vi "MSEncoder SubVI WfmCodeGen_AuxScan.vi"(0 "MSEncoder in":refnum<class "MSEncoder.lvclass">=refnum, 1 "Scan time":ext=0.1, 2 "Pulse1 Amp":ext=-0.55, 3 "mz0":ext=608.9080247841045691, 4 "Amp ramp rate":ext=-0.0, 5 "Pulse2 Amp":ext=0.55, 6 "Start conj #":u32, 7 "Scan rate":ext=-0.0, 8 "Beta scale":ext=1.0, 9 "Wfm type":u64=2, 10 "MathieuEqParame":T1={"mz(Th)"=608.9080247841045691, "Amp(V)"=300.0, "Freq(Hz)"=301269.66536045074, "Beta"=0.39999999999999986, "r_0 (mm)"=10.0, "z_0 (mm)"=7.07106781187} {"Freq(Hz)" format="%#_2g"; "Amp(V)" format="%#.2g"; "mz(Th)" format="%#.2g"}, 11 "Amp0":ext, 13 "TotalAuxCyc#":ext=1.0) -> (17 "WfmCode":u64[](array[numeric]), 19 "error out":errorcluster)   [LabVIEW 2018, in "MSEncoder.lvclass"]
uses:
  MSEncoder.lvclass
  PublicSubVI/Ctl/MathieuEqParam.ctl
  MSEncoder.lvclass/MSEncoder.ctl
panel:
  in  "High Res":bool
  out "start conj":u64[](array[numeric])
  out "RF Cycle":u64[](array[numeric])
  out "decimated array":u64[](array[numeric])
  in  "Interrupt":bool
  out "Aux Scan":cluster{"Scan time":ext, "Actual Freq":dbl}[](graph)
  out "Progress":dbl(slide)=-1.0 scale=0.0..0.1
  out "PriRF.Decyc":u32=32348584
  out "CrntConj.CycDiff":u64[](array[numeric])=[2147483648]
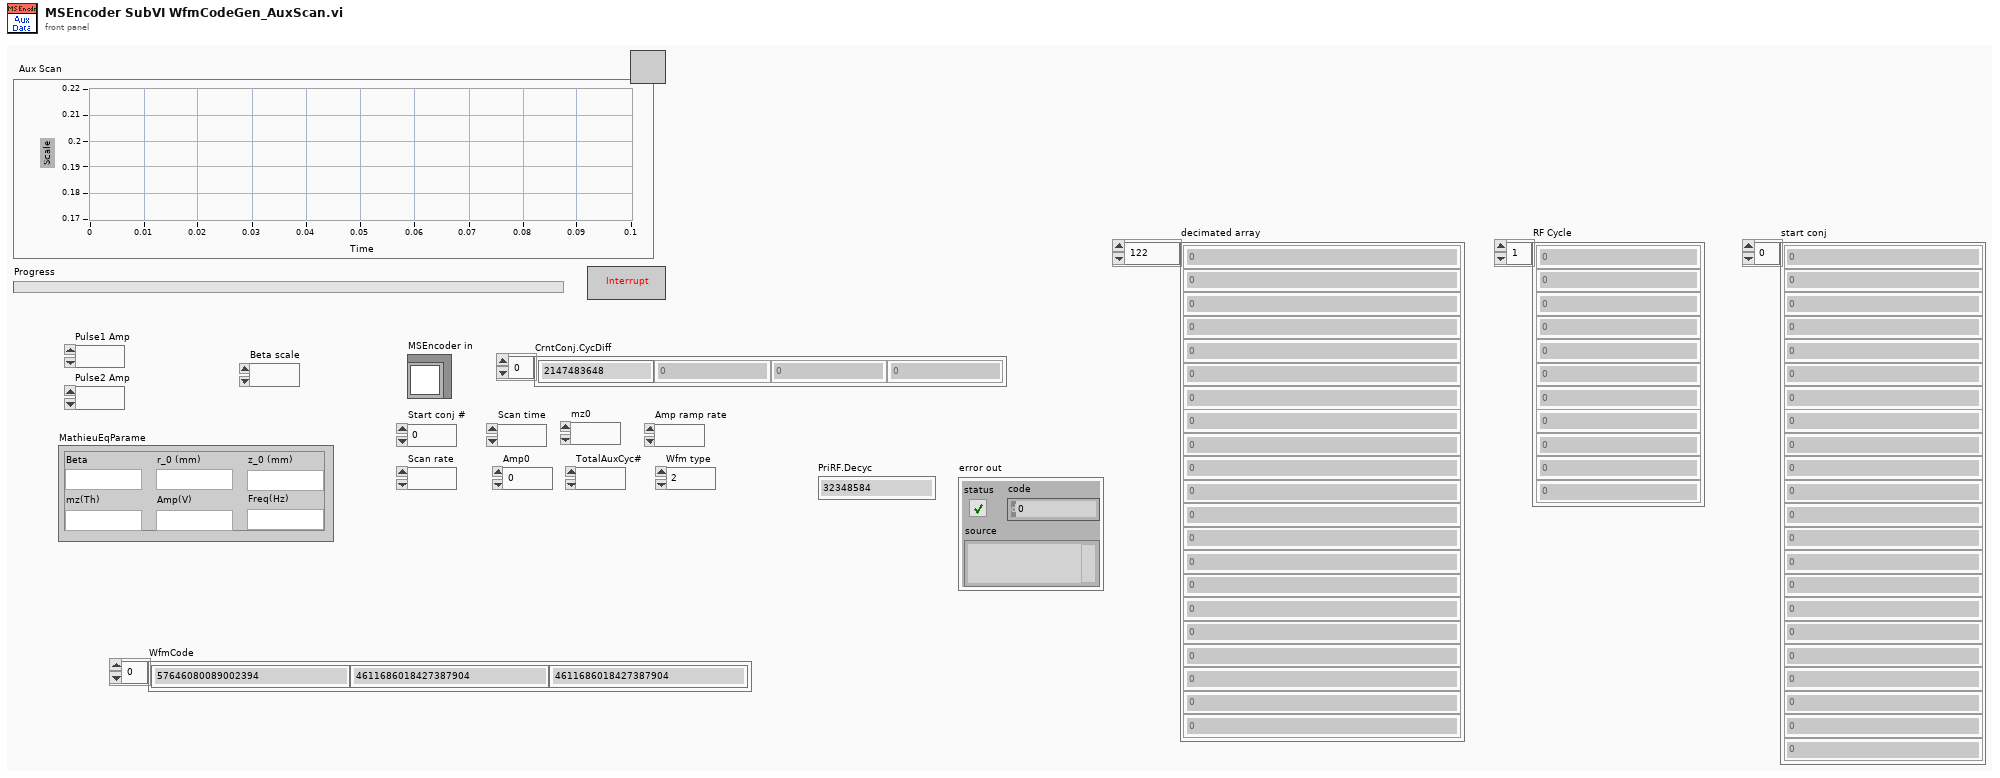
[diagram p1: front panel]
types:
  T1 = typedef "MathieuEqParam.ctl" = cluster{"mz(Th)":ext, "Amp(V)":ext, "Freq(Hz)":ext, "Beta":ext, "r_0 (mm)":ext, "z_0 (mm)":ext}
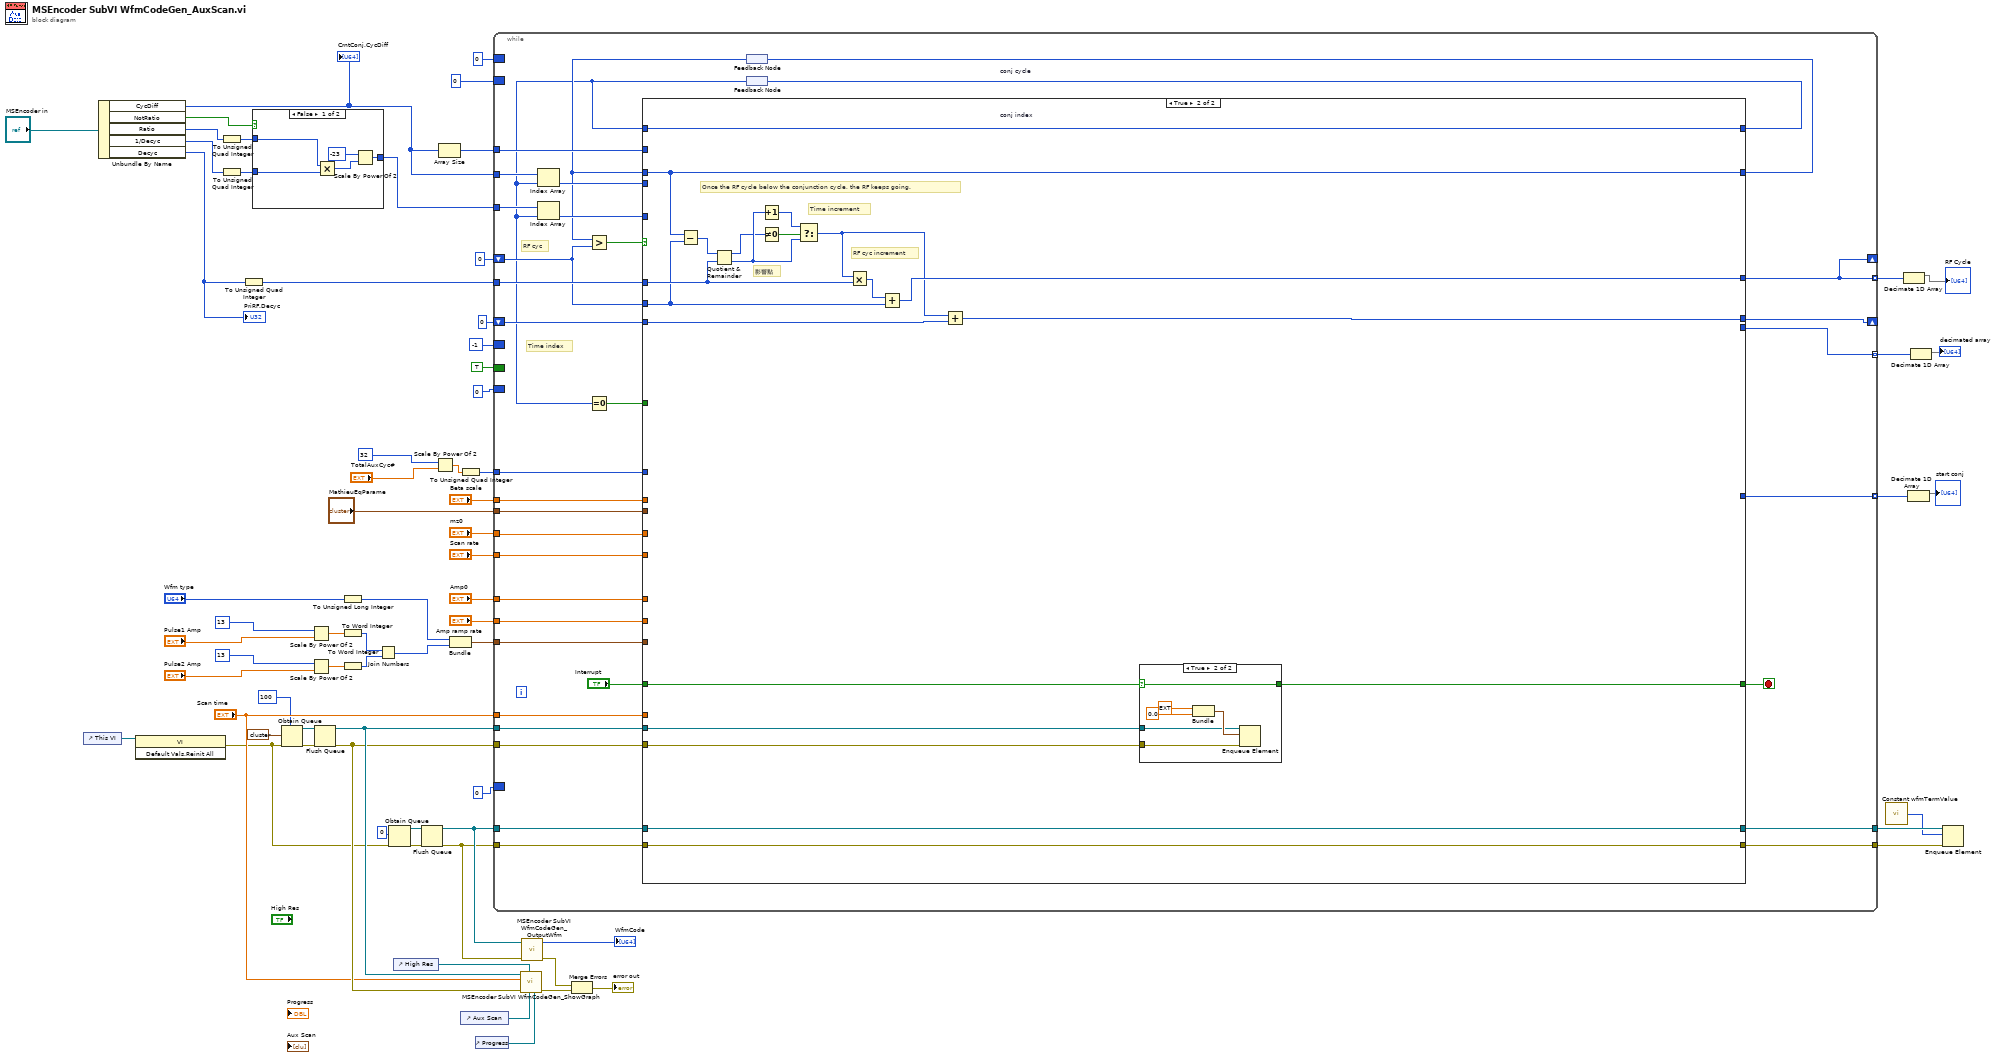
[diagram p0: block diagram]
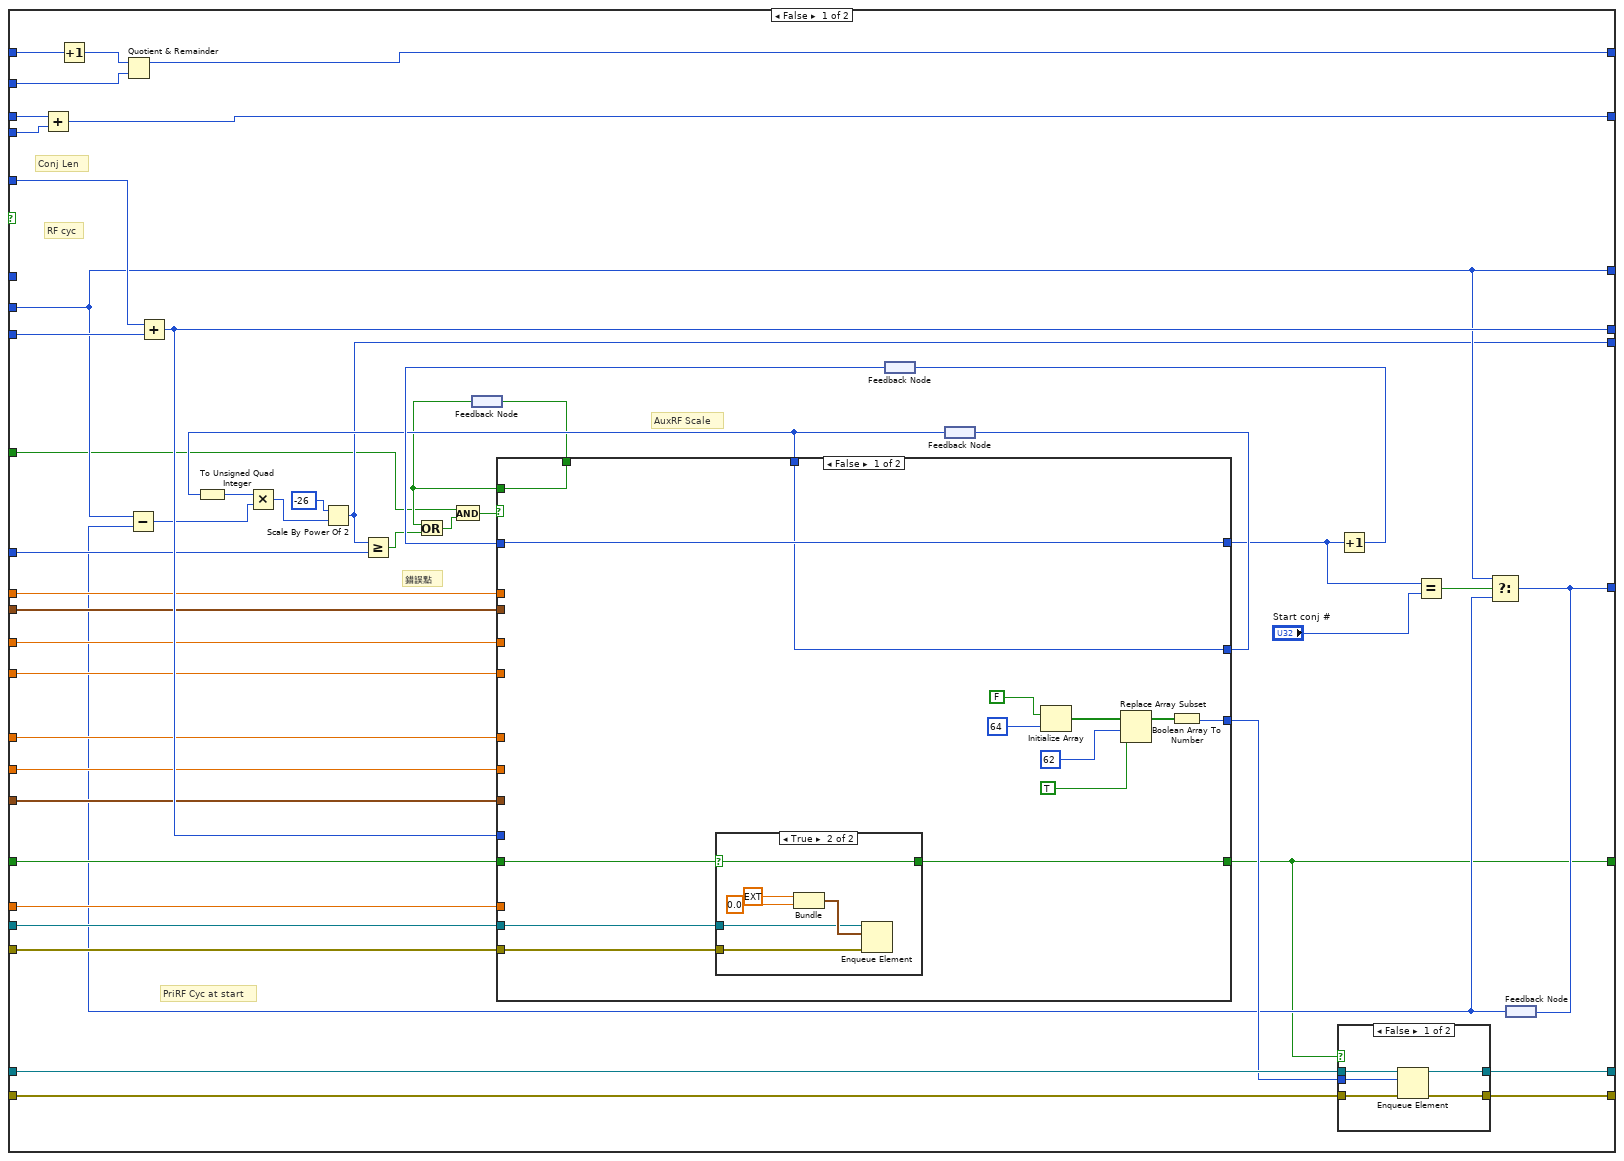
[diagram p3: hidden frame]
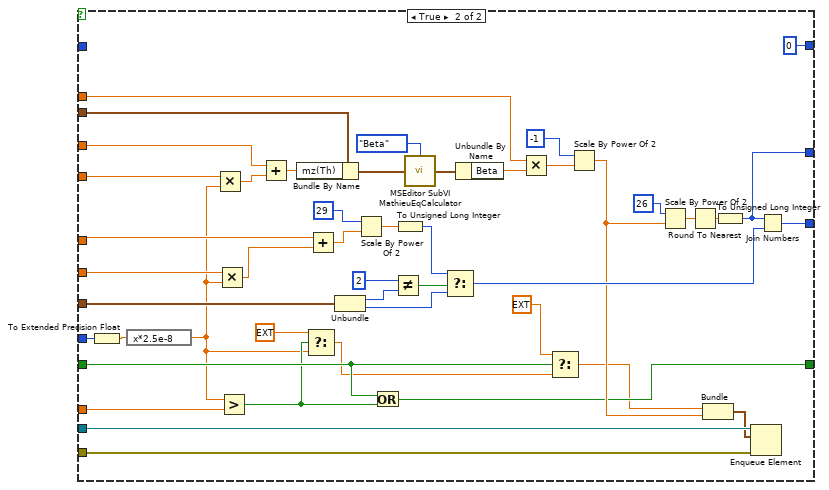
[diagram p6: hidden frame]
diagram:
  n1 = control-ref of="This VI"() -> (w9:refnum<vi>)
  n2 = Unbundle By Name("MSEncoder in") -> ("CycDiff"=w56:u64[], "NotRatio"=w40:bool, "Ratio"=w68:u16[], "1/Decyc"=w69:u32, "Decyc"=w71:u32)
  "CrntConj.CycDiff" <- w56
  "PriRF.Decyc" <- w71
  n3 = invoke class="VI" method="Default Vals.Reinit All"(reference=w9) -> (error out=w8:errorcluster)  [unwired: 2 in, 2 out]
  n4 = To Unsigned Quad Integer(1:w68) -> (0:w70:u64[])
  n5 = To Unsigned Quad Integer(1:w69) -> (0:w54:u64)
  n6 = To Unsigned Quad Integer(1:w71) -> (0:w53:u64)
  n7 = case shown="False" w40 {
    tunnel: w70 -> [w74 w77]
    tunnel: [w73 w77] -> w57
    tunnel: w54 -> [w72 _]
    frame False {
      n8 = Multiply(x=w74, y=w72) -> (x*y=w75:u64[])
      n9 = Scale By Power Of 2(n=i16 -23, x=w75) -> (x*2^n=w73:u64[])
    }
    frame True {
    }
  }
  n10 = Obtain Queue(max queue size (-1, unlimited)=100, element data type=cluster{"Scan time":ext, "Actual Freq":ext} {"Scan time"=0.0, "Actual Freq"=0.0} ("output cluster"), error in (no error)=w8) -> (queue out=w23:refnum<queue>, error out=w24:errorcluster)  [unwired: 2 in, 1 out]
  n11 = Scale By Power Of 2(n=i16 13, x="Pulse1 Amp") -> (x*2^n=w63:ext)
  n12 = Scale By Power Of 2(n=i16 13, x="Pulse2 Amp") -> (x*2^n=w64:ext)
  n13 = Flush Queue(queue=w23, error in (no error)=w24) -> (queue out=w17:refnum<queue>, error out=w16:errorcluster)  [unwired: 1 out]
  n14 = To Unsigned Long Integer(number="Wfm type") -> (unsigned 32bit integer=w44:u32)
  n15 = To Word Integer(number=w63) -> (16bit integer=w65:i16)
  n16 = To Word Integer(number=w64) -> (16bit integer=w66:i16)
  n17 = Join Numbers(hi=w65, lo=w66) -> ((hi.lo)=w45:u32)
  n18 = Obtain Queue(element data type=u64 0, error in (no error)=w8) -> (queue out=w26:refnum<queue>, error out=w25:errorcluster)  [unwired: 3 in, 1 out]
  n19 = control-ref of="High Res"() -> (w1:refnum<vi>)
  n20 = Flush Queue(queue=w26, error in (no error)=w25) -> (queue out=w19:refnum<queue>, error out=w18:errorcluster)  [unwired: 1 out]
  n21 = Scale By Power Of 2(n=i16 32, x="TotalAuxCyc#") -> (x*2^n=w34:ext)
  n22 = Array Size(array=w56) -> (size(s)=w55:i32)
  n23 = Bundle(w44, w45) -> (w43:cluster{u32, u32})  [unwired: 1 in]
  n24 = To Unsigned Quad Integer(1:w34) -> (0:w33:u64)
  n25 = control-ref of="Aux Scan"() -> (w13:refnum<vi>)
  n26 = control-ref of="Progress"() -> (w12:refnum<vi>)
  n27 = while {
    tunnel: w56 -> [w112]
    border: u64 0 -> [_]
    tunnel: w55 -> [w108]
    tunnel: "mz0" -> [w106]
    tunnel: w57 -> [w111]
    tunnel: "Scan time" -> [w107]
    tunnel: "MathieuEqParame" -> [w105]
    tunnel: w17 -> [w102]
    tunnel: w16 -> [w101]
    border: 0 -> [_]
    tunnel: w53 -> [w104]
    tunnel: "Scan rate" -> [w100]
    tunnel: "Beta scale" -> [w99]
    tunnel: "Amp0" -> [w98]
    tunnel: "Amp ramp rate" -> [w97]
    tunnel: w43 -> [w96]
    border: u32 0 -> [_]
    shift-right: [w81] -> _
    shift-left: u64 0 -> [w95]
    shift-right: [w79] -> _
    shift-left: u64 0 -> [w93]
    tunnel: w33 -> [w89]
    border: u64 0 -> [_]
    border: -1 -> [_]
    border: TRUE -> [_]
    tunnel: w19 -> [w88]
    tunnel: w18 -> [w87]
    tunnel: [w86] -> w28
    tunnel: [w85] -> w27
    tunnel: [w82] -> w7 mode=indexing
    tunnel: [w79] -> w5 mode=indexing
    tunnel: [w78] -> w4 mode=indexing
    stop <- w103 stop-if-true
    # "RF cyc"
    # "Time index"
    n28 = feedback #1 "conj cycle"() -> (w94:u64)
    n29 = Greater?(x=w94, y=w93) -> (0:w92:bool)
    n30 = feedback #2 "conj index"() -> (w91:i32)
    n31 = Index Array(array=w112, index=w91) -> (element=w109:u64)
    n32 = Index Array(array=w111, index=w91) -> (element=w110:u64)
    n33 = Equal To 0?(x=w91) -> (x = 0?=w90:bool)
    n34 = case shown="True" w92 {
      tunnel: w110 -> [w146 _]
      tunnel: w109 -> [w159 _]
      tunnel: w94 -> [w158 w251]
      tunnel: w104 -> [_ w249]
      tunnel: w93 -> [w138 w237]
      tunnel: w108 -> [w155 _]
      tunnel: [w157 w251] -> w80
      tunnel: w91 -> [w152 w255]
      tunnel: [w154 w255] -> w83
      tunnel: [w160 w236] -> w81
      tunnel: w95 -> [w153 w254]
      tunnel: [w138 w252] -> w79
      tunnel: w107 -> [w151 _]
      tunnel: w106 -> [w150 _]
      tunnel: w105 -> [w149 _]
      tunnel: [w113 w243] -> w103
      tunnel: w102 -> [w148 w241]
      tunnel: w101 -> [w147 w240]
      tunnel: w100 -> [w145 _]
      tunnel: w99 -> [w144 _]
      tunnel: w98 -> [w143 _]
      tunnel: w97 -> [w142 _]
      tunnel: w96 -> [w141 _]
      tunnel: w90 -> [w119 _]
      tunnel: w89 -> [w123 _]
      tunnel: w88 -> [w130 w245]
      tunnel: w87 -> [w129 w244]
      tunnel: [w128 w245] -> w86
      tunnel: [w127 w244] -> w85
      tunnel: "Interrupt" -> [w126 w242]
      tunnel: [w124 _] -> w82
      tunnel: [w121 _] -> w78
      frame False {
        # "錯誤點"
        # "Conj Len"
        # "RF cyc"
        # "AuxRF Scale"
        # "PriRF Cyc at start"
        n35 = Add(x=w158, y=w159) -> (x+y=w157:u64)
        n36 = Increment(x=w152) -> (x+1=w156:i32)
        n37 = Quotient & Remainder(x=w156, y=w155) -> (x-y*floor(x/y)=w154:i32)  [unwired: 1 out]
        n38 = Add(x=w146, y=w153) -> (x+y=w160:u64)
        n39 = feedback #3() -> (w120:bool)
        n40 = feedback #4() -> (w161:i32)
        n41 = feedback #5() -> (w136:u32)
        n42 = To Unsigned Quad Integer(1:w136) -> (0:w135:u64)
        n43 = feedback #6() -> (w114:u64)
        n44 = Subtract(x=w138, y=w114) -> (x-y=w137:u64)
        n45 = Multiply(x=w135, y=w137) -> (x*y=w133:u64)
        n46 = Scale By Power Of 2(n=i16 -26, x=w133) -> (x*2^n=w124:u64)
        n47 = Greater Or Equal?(x=w124, y=w123) -> (x >= y?=w118:bool)
        n48 = Or(x=w120, y=w118) -> (x .or. y?=w132:bool)
        n49 = And(x=w119, y=w132) -> (x .and. y?=w140:bool)
        n50 = case shown="False" w140 {
          tunnel: w149 -> [_ w223]
          tunnel: w150 -> [_ w224]
          tunnel: w151 -> [_ w235]
          tunnel: [w176 w215] -> w125
          tunnel: [w169 w198] -> w113
          tunnel: w148 -> [w171 w234]
          tunnel: w147 -> [w170 w233]
          tunnel: w145 -> [_ w231]
          tunnel: w144 -> [_ w227]
          tunnel: w143 -> [_ w219]
          tunnel: w142 -> [_ w221]
          tunnel: w141 -> [_ w214]
          tunnel: [w174 w199] -> w122
          tunnel: w161 -> [w175 _]
          tunnel: [w175 0] -> w116
          tunnel: w160 -> [_ w207]
          tunnel: w136 -> [w174 _]
          tunnel: w120 -> [w173 _]
          tunnel: [w173 _] -> w131
          tunnel: w126 -> [w172 w197]
          frame False {
            n51 = case shown="True" w172 {
              selector: w172 -> [w183 w184]
              tunnel: w171 -> [_ w186]
              tunnel: w170 -> [_ w185]
              tunnel: [w183 w184] -> w169
              frame False {
              }
              frame True {
                n52 = Bundle(ext -1.0, 0.0) -> (w189:cluster{ext, dbl})  [unwired: 1 in]
                n53 = Enqueue Element(queue=w186, element=w189, error in (no error)=w185) -> ()  [unwired: 1 in, 3 out]
              }
            }
            n54 = Initialize Array(FALSE, 64 ("dimension size")) -> (w180:bool[])
            n55 = Replace Array Subset(array=w180, new element=TRUE, index=62) -> (w177:bool[])
            n56 = Boolean Array To Number(Boolean array=w177) -> (number=w176:u64)
          }
          frame True {
            n57 = To Extended Precision Float(1:w207) -> (0:w201:ext)
            n58 = expression code="x*2.5e-8"(w201) -> (w190:ext)
            n59 = Multiply(x=w231, y=w190) -> (x*y=w225:ext)
            n60 = Multiply(x=w221, y=w190) -> (x*y=w220:ext)
            n61 = Greater?(x=w190, y=w235) -> (0:w193:bool)
            n62 = Add(x=w224, y=w225) -> (x+y=w226:ext)
            n63 = Bundle By Name(cluster=w223, "mz(Th)"=w226) -> (w222:T1)
            n64 = Select(t=ext -2.0, s=w193, f=w190) -> (s? t:f=w191:ext)
            n65 = Add(x=w219, y=w220) -> (x+y=w216:ext)
            n66 = Unbundle(w214) -> (w213:u32, w209:u32)
            n67 = Scale By Power Of 2(n=i16 29, x=w216) -> (x*2^n=w217:ext)
            n68 = Or(x=w197, y=w193) -> (x .or. y?=w198:bool)
            n69 = Not Equal?(x=u32 2, y=w213) -> (x != y?=w211:bool)
            n70 = To Unsigned Long Integer(number=w217) -> (unsigned 32bit integer=w210:u32)
            n71 = call "MSEditor SubVI MathieuEqCalculator.vi"("Target (Freq)"=enum16{"m/z", "Volt", "Freq", "Beta"}."Beta", "Parametres in"=w222) -> ("Parametres out"=w229:T1)  [unwired: 2 in]
            n72 = Select(t=w210, s=w211, f=w209) -> (s? t:f=w208:u32)
            n73 = Unbundle By Name(w229) -> ("Beta"=w203:ext)
            n74 = Multiply(x=w227, y=w203) -> (x*y=w202:ext)
            n75 = Select(t=ext -1.0, s=w197, f=w191) -> (s? t:f=w195:ext)
            n76 = Scale By Power Of 2(n=i16 -1, x=w202) -> (x*2^n=w200:ext)
            n77 = Scale By Power Of 2(n=i16 26, x=w200) -> (x*2^n=w205:ext)
            n78 = Round To Nearest(number=w205) -> (nearest integer value=w204:ext)
            n79 = Bundle("t"=w195, w200) -> (w232:cluster{"t":ext, ext})  [unwired: 1 in]
            n80 = To Unsigned Long Integer(number=w204) -> (unsigned 32bit integer=w199:u32)
            n81 = Enqueue Element(queue=w234, element=w232, error in (no error)=w233) -> ()  [unwired: 1 in, 3 out]
            n82 = Join Numbers(hi=w199, lo=w208) -> ((hi.lo)=w215:u64)
          }
        }
        n83 = feedback-in #3(w131) -> ()
        n84 = feedback-in #5(w122) -> ()
        n85 = case shown="False" w113 {
          tunnel: w130 -> [w166 w168]
          tunnel: w129 -> [w165 w167]
          tunnel: [w164 w168] -> w128
          tunnel: [w163 w167] -> w127
          tunnel: w125 -> [w162 _]
          frame False {
            n86 = Enqueue Element(queue=w166, element=w162, error in (no error)=w165) -> (queue out=w164:refnum<queue>, error out=w163:errorcluster)  [unwired: 1 in, 1 out]
          }
          frame True {
          }
        }
        n87 = Increment(x=w116) -> (x+1=w139:i32)
        n88 = feedback-in #4(w139) -> ()
        n89 = Equal?(x=w116, y="Start conj #") -> (x = y?=w115:bool)
        n90 = Select(t=w138, s=w115, f=w114) -> (s? t:f=w121:u64)
        n91 = feedback-in #6(w121) -> ()
      }
      frame True {
        # "影響點"
        # "Time increment"
        # "RF cyc increment"
        # "Once the RF cycle below the conjunction cycle, the RF keeps going."
        n92 = Subtract(x=w251, y=w237) -> (x-y=w250:u64)
        n93 = Quotient & Remainder(x=w250, y=w249) -> (x-y*floor(x/y)=w238:u64, floor(x/y)=w247:u64)
        n94 = Increment(x=w247) -> (x+1=w246:u64)
        n95 = Not Equal To 0?(x=w238) -> (x != 0?=w248:bool)
        n96 = Select(t=w246, s=w248, f=w247) -> (s? t:f=w239:u64)
        n97 = Multiply(x=w239, y=w249) -> (x*y=w253:u64)
        n98 = Add(x=w253, y=w237) -> (x+y=w252:u64)
        n99 = Add(x=w239, y=w254) -> (x+y=w236:u64)
        n100 = case shown="True" w242 {
          selector: w242 -> [w256 w257]
          tunnel: w241 -> [_ w259]
          tunnel: w240 -> [_ w258]
          tunnel: [w256 w257] -> w243
          frame False {
          }
          frame True {
            n101 = Bundle(ext -1.0, 0.0) -> (w262:cluster{ext, dbl})  [unwired: 1 in]
            n102 = Enqueue Element(queue=w259, element=w262, error in (no error)=w258) -> ()  [unwired: 1 in, 3 out]
          }
        }
      }
    }
    n103 = feedback-in #1(w80) -> ()
    n104 = feedback-in #2(w83) -> ()
  }
  n105 = call "MSEncoder SubVI WfmCodeGen_ShowGraph.vi"("progress refnum"=w12, "system graph refnum"=w13, "Graph Display"=w1, "error in (no error)"=w16, "X Scale.Range:Maximum"="Scan time", "Display queue in"=w17) -> ("error out"=w20:errorcluster)  [unwired: 5 in]
  n106 = call "MSEncoder SubVI WfmCodeGen_OutputWfm.vi"("error in (no error)"=w18, "calc wfm queue"=w19) -> ("error out"=w21:errorcluster, "WfmCode"=→"WfmCode":u64[])  [unwired: 8 in]
  n107 = Merge Errors(w21, w20) -> (→"error out":errorcluster)
  n108 = call "Constant wfmTermValue.vi"() -> ("wfm end value"=w22:u64)
  n109 = Decimate 1D Array(w5) -> (→"RF Cycle":u64[])  [unwired: 1 out]
  n110 = Decimate 1D Array(w4) -> (→"start conj":u64[])  [unwired: 1 out]
  n111 = Decimate 1D Array(w7) -> (→"decimated array":u64[])  [unwired: 1 out]
  n112 = Enqueue Element(queue=w28, element=w22, error in (no error)=w27) -> ()  [unwired: 1 in, 3 out]
